vi "Desktop Main.vi"() -> ()   [LabVIEW 2014]
uses:
  <resource>/objmgr/ni.dex.rc
  <vilib>/measure/NI_MAPro.lvlib
  <vilib>/sound2/lvsound2.llb/Sound Data Format.ctl
  <vilib>/sound2/lvsound2.llb/Sound File Write (I16).vi
  <vilib>/sound2/lvsound2.llb/Sound File Write Open.vi
  <vilib>/measure/maspectr.llb/FFT Power Spectrum and PSD for N Chan.vi
panel:
  in  "OP Mic On":bool
  in  "Record Button":bool
  out "Record Counter":dbl
  in  "Noise Sample Length":dbl
  out "Noise sample path":path
  out "Audio Signal":waveform(i16)[](graph)
  out "Connected?":bool
  in  "Target IP Address":string="172.22.11.2"
  in  "Stop":bool
  out "Frequency Spectrum":cluster{"f0":dbl, "df":dbl, "magnitude":dbl[]}[](graph)
  # "Overview: This sample project shows how to retrieve and process data from NI myRIO using network streams.\nRequirements: LabVIEW FPGA Module, Network Streams software on the NI myRIO RT target. \nInstructions:\n1. Run the RT Main.vi on the myRIO target.\n2. Run the Desktop Main.vi.  \n3. Click Record button to save the signal to .wav file."
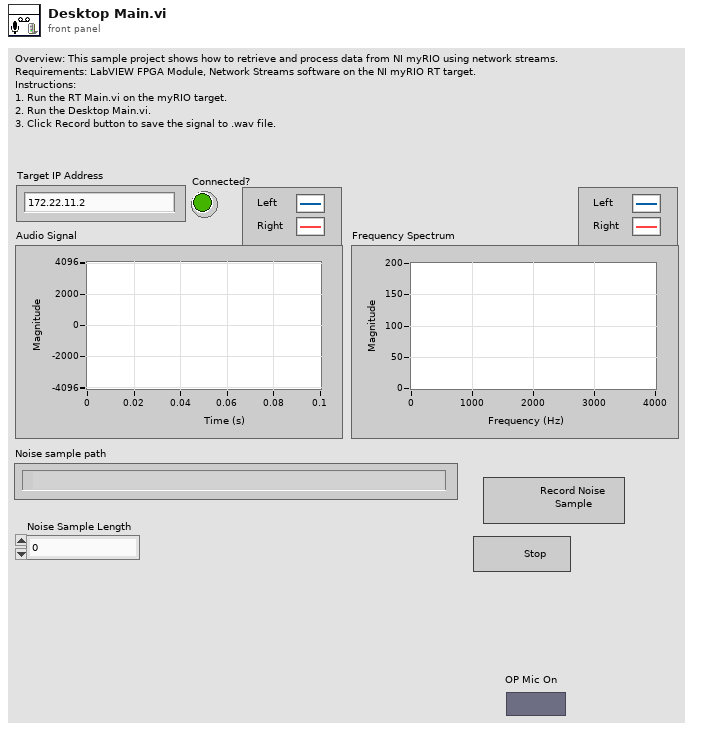
[diagram p1: front panel]
types:
  T1 = typedef "Sound Data Format.ctl" = cluster{"sample rate (S/s)":dbl, "number of channels":i32, "bits per sample":i32}
  T2 = typedef "Sound File Refnum.ctl" = refnum<file>
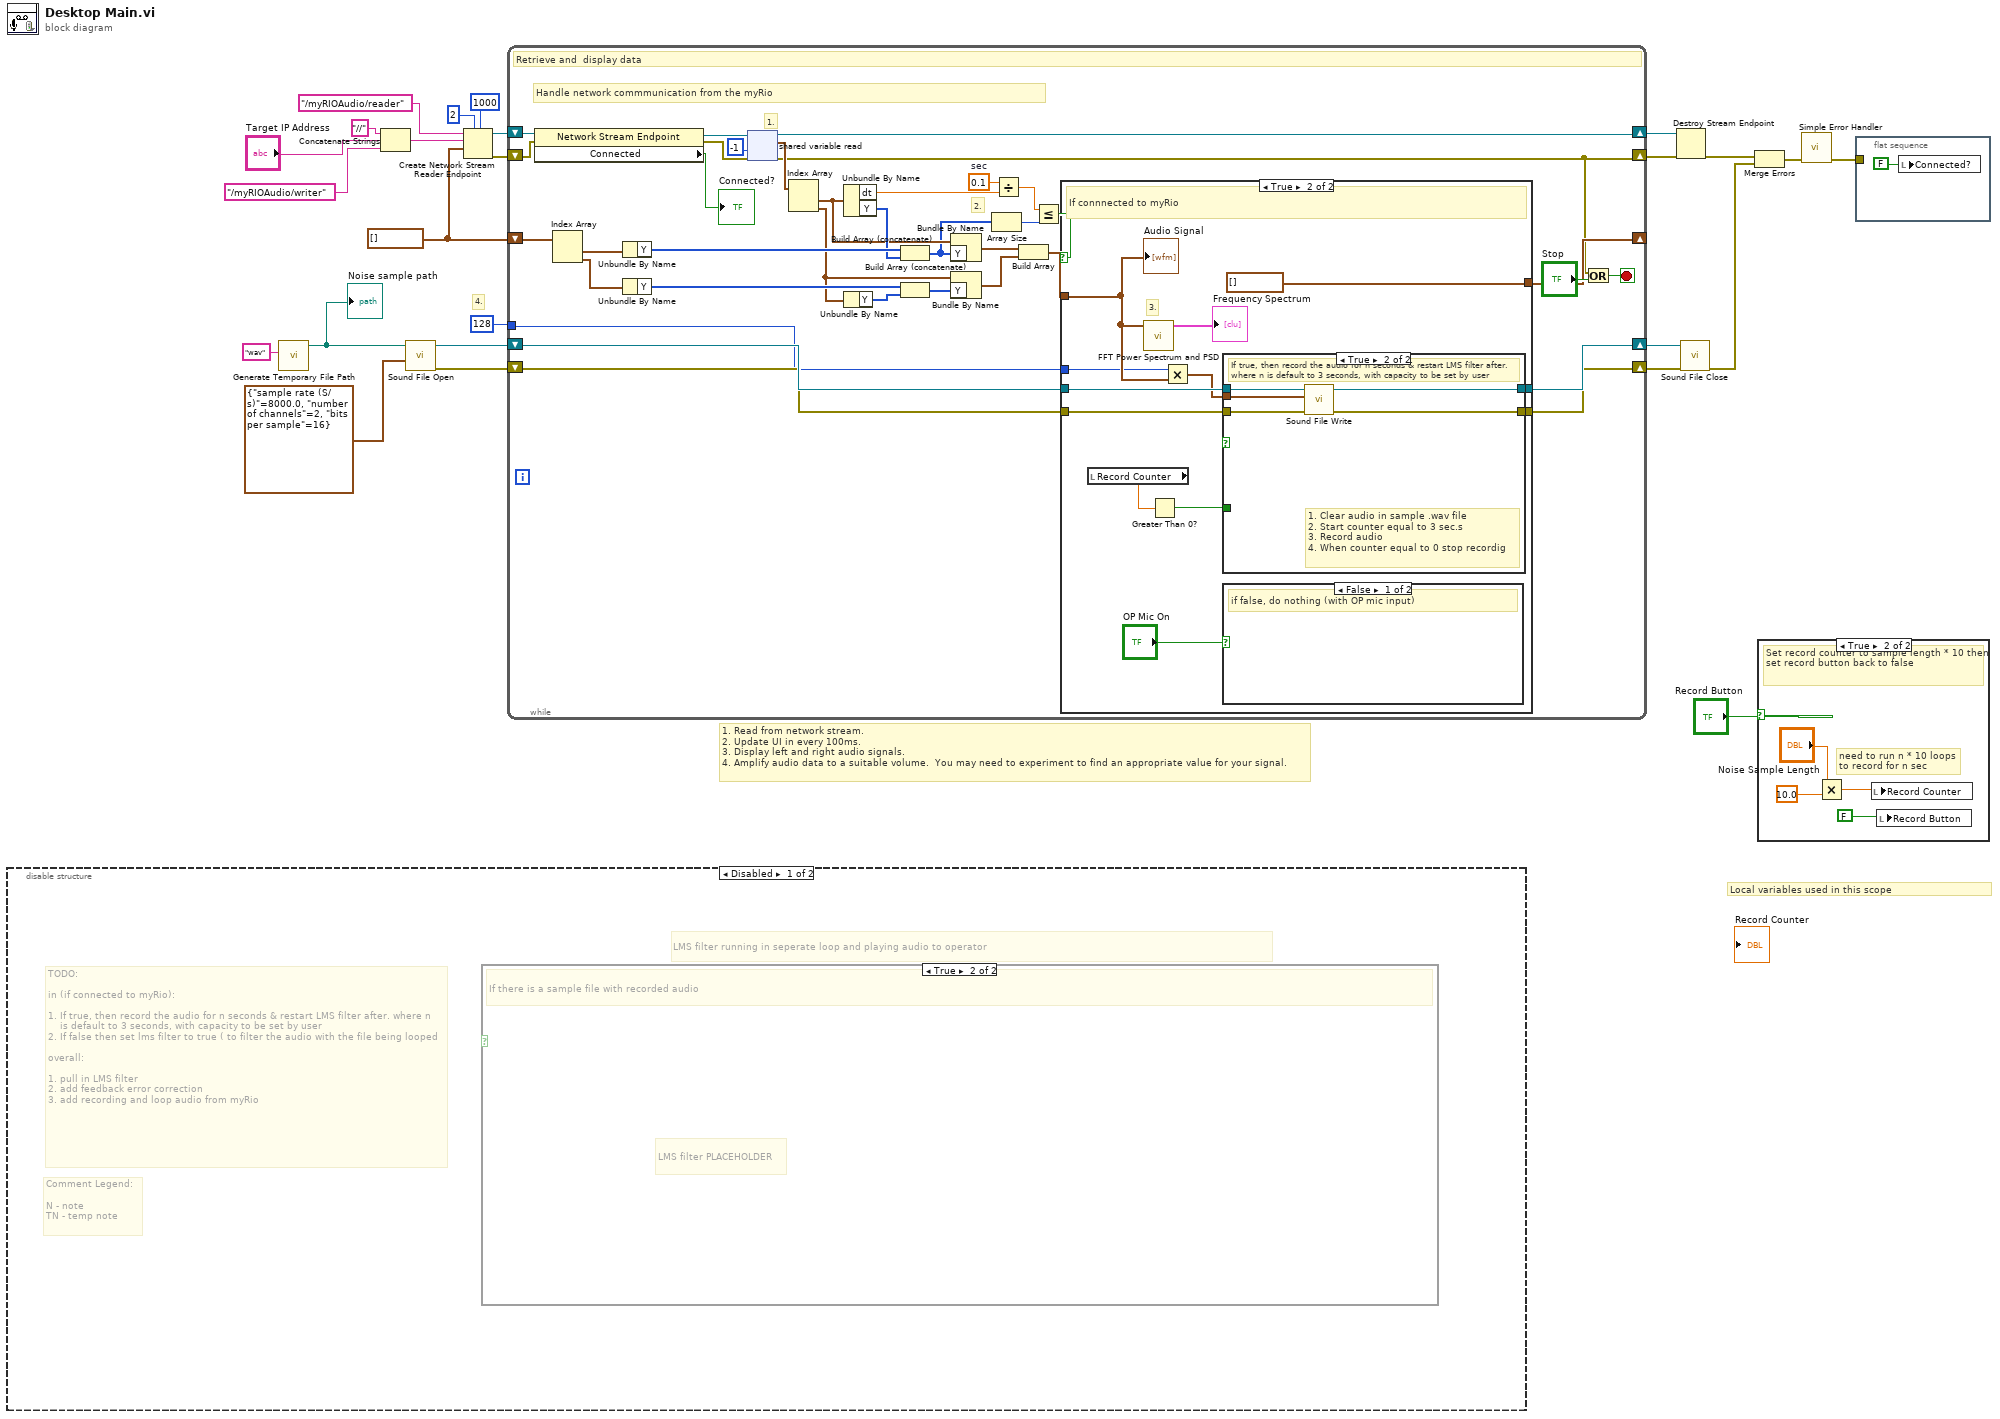
[diagram p0: block diagram]
diagram:
  w5 = waveform(i16)[] []
  # "Local variables used in this scope"
  # "4."
  # "1. Read from network stream.\n2. Update UI in every 100ms.\n3. Display left and right audio signals.\n4. Amplify audio data to a suitable volume.  You may need to experiment to find an appropriate value for your signal."
  n1 = disable-structure shown="Disabled" {
    frame Disabled {
      # "Comment Legend:\n\nN - note\nTN - temp note"
      # "TODO:\n\nin (if connected to myRio):\n\n1. If true, then record the audio for n seconds & restart LMS filter after. where n \n    is default to 3 seconds, with capacity to be set by user\n2. If false then set lms filter to true ( to filter the audio with the file being looped\n\noverall:\n\n1. pull in LMS filter\n2. add feedback error correction\n3. add recording and loop audio from myRio"
      # "LMS filter running in seperate loop and playing audio to operator"
      n2 = case shown="True" {
        selector: _ -> [_ _]
        frame False {
          # "If there is no recorded audio"
        }
        frame True {
          # "LMS filter PLACEHOLDER"
          # "If there is a sample file with recorded audio"
        }
      }
    }
    frame Enabled {
    }
  }
  n3 = call <vilib>:"Generate Temporary File Path.vi"("Temporary File Extension (tmp)"="wav") -> ("Unique Temporary File Path"=w8:path)  [unwired: 9 in, 1 out]
  "Noise sample path" <- w8
  n4 = Concatenate Strings("//" ("reader url"), "Target IP Address", "/myRIOAudio/writer") -> (w17:string)
  n5 = call-poly <vilib>:"Sound File Open.vi"("sound format"=T1 {"sample rate (S/s)"=8000.0, "number of channels"=2, "bits per sample"=16}, "path"=w8) -> ("error out"=w11:errorcluster, "sound file refnum"=w13:T2)  [unwired: 8 in]
  n6 = Create Network Stream Reader Endpoint(5:1000 ("timeout in ms (-1)"), 7:2 ("reader buffer size"), 9:w5, 10:w17, 11:"/myRIOAudio/reader" ("writer name")) -> (0:w23:errorcluster, 3:w24:refnum<k21>)  [unwired: 2 in]
  n7 = while {
    shift-right: [w59] -> w22
    shift-left: w24 -> [w58]
    shift-right: [w44] -> w21
    shift-left: w23 -> [w55]
    shift-right: [w49] -> _
    shift-left: w5 -> [w51]
    shift-right: [w42] -> w12
    shift-left: w13 -> [w43]
    shift-right: [w40] -> w10
    shift-left: w11 -> [w41]
    tunnel: i16 128 -> [w39]
    stop <- w60 stop-if-true
    w47 = 0.1  # sec
    # "Handle network commmunication from the myRio"
    # "2."
    # "1."
    # "Retrieve and  display data"
    n8 = property class="Network Stream Endpoint"(reference=w58, error in=w55) -> (reference out=w56:refnum<k21>, error out=w54:errorcluster, "Connected"=→"Connected?":bool)
    n9 = Index Array(array=w51) -> (element #1=w38:waveform(i16), element #2=w37:waveform(i16))  [unwired: 2 in]
    n10 = Unbundle By Name(w38) -> ("Y"=w36:i16[])
    n11 = Unbundle By Name(w37) -> ("Y"=w34:i16[])
    n12 = shared-variable-read(w56, w54, -1 ("timeout ms (-1)")) -> (w59:refnum<k21>, w44:errorcluster, w52:waveform(i16)[])  [unwired: 1 out]
    n13 = Index Array(array=w52) -> (element #1=w32:waveform(i16), element #2=w29:waveform(i16))  [unwired: 2 in]
    n14 = Unbundle By Name(w32) -> ("dt"=w48:dbl, "Y"=w35:i16[])
    n15 = Unbundle By Name(w29) -> ("Y"=w33:i16[])
    n16 = Build Array (concatenate)(w36, w35) -> (w26:i16[])
    n17 = Build Array (concatenate)(w34, w33) -> (w28:i16[])
    n18 = Bundle By Name(cluster=w32, "Y"=w26) -> (w30:waveform(i16))
    n19 = Bundle By Name(cluster=w29, "Y"=w28) -> (w27:waveform(i16))
    n20 = Array Size(array=w26) -> (size(s)=w31:i32)
    n21 = Divide(x=w47, y=w48) -> (x/y=w45:dbl)
    n22 = Build Array(w30, w27) -> (w50:waveform(i16)[])
    n23 = Less Or Equal?(x=w45, y=w31) -> (x <= y?=w46:bool)
    n24 = case shown="True" w46 {
      tunnel: w50 -> [w64 w71]
      tunnel: [w64 waveform(i16)[] []] -> w49
      tunnel: w43 -> [w63 w75]
      tunnel: [w63 w74] -> w42
      tunnel: w41 -> [w62 w72]
      tunnel: [w62 w73] -> w40
      tunnel: w39 -> [_ w69]
      frame False {
      }
      frame True {
        # "3."
        # "If connnected to myRio"
        n25 = local read "Record Counter"() -> (w66:dbl)
        n26 = call-poly <vilib>:"FFT Power Spectrum and PSD.vi"("time signals"=w71) -> ("Power Spectrum / PSD"=→"Frequency Spectrum":cluster{"f0":dbl, "df":dbl, "magnitude":dbl[]}[])  [unwired: 7 in, 3 out]
        n27 = Greater Than 0?(x=w66) -> (x > 0?=w67:bool)
        n28 = Multiply(x=w69, y=w71) -> (x*y=w70:waveform(i16)[])
        n29 = case shown="True" {
          selector: _ -> [_ _]
          tunnel: w75 -> [w78 w83]
          tunnel: [w78 w82] -> w74
          tunnel: [w77 w81] -> w73
          tunnel: w70 -> [_ w80]
          tunnel: w72 -> [w77 w79]
          tunnel: w67 -> [_ _]
          frame False {
            # "Pass incoming audio to LMS filter"
          }
          frame True {
            # "1. Clear audio in sample .wav file\n2. Start counter equal to 3 sec.s\n3. Record audio \n4. When counter equal to 0 stop recordig"
            # "If true, then record the audio for n seconds & restart LMS filter after. where n is default to 3 seconds, with capacity to be set by user"
            n30 = call-poly <vilib>:"Sound File Write.vi"("error in (no error)"=w79, "data"=w80, "sound file refnum"=w83) -> ("error out"=w81:errorcluster, "sound file refnum out"=w82:T2)  [unwired: 7 in]
          }
        }
        n31 = case shown="False" "OP Mic On" {
          frame False {
            # "if false, do nothing (with OP mic input)"
          }
          frame True {
            # "1. Send signal to my rio to quiet or \n    mute audio on myRio\n2. Send audio to the myRio"
            # "if true, quiet myRio & send audio"
          }
        }
        "Audio Signal" <- w71
      }
    }
    n32 = Or(x=w44, y="Stop") -> (x .or. y?=w60:bool)
  }
  n33 = Destroy Stream Endpoint(8:w21, 11:w22) -> (0:w15:errorcluster)
  n34 = call <vilib>:"Sound File Close.vi"("error in (no error)"=w10, "sound file refnum"=w12) -> ("error out"=w2:errorcluster)  [unwired: 9 in]
  n35 = Merge Errors(w15, w2) -> (w3:errorcluster)
  n36 = case shown="True" "Record Button" {
    frame False {
    }
    frame True {
      # "need to run n * 10 loops\nto record for n sec"
      # "Set record counter to sample length * 10 then set record button back to false"
      n37 = Multiply(x="Noise Sample Length", y=10.0) -> (x*y=w86:dbl)
      n38 = local write "Record Counter"(w86) -> ()
      n39 = local write "Record Button"(FALSE) -> ()
    }
  }
  n40 = call <vilib>:"Simple Error Handler.vi"("error in (no error)"=w3) -> ("error out"=w4:errorcluster)  [unwired: 4 in, 4 out]
  n41 = flat-sequence {
    tunnel: w4 -> [_]
    frame #0 {
      n42 = local write "Connected?"(FALSE ("Connected?")) -> ()
    }
  }
